vi "RT - Initialize Valves.vi"(8 "error in":errorcluster) -> (0 "error out":errorcluster)   [LabVIEW 2018]
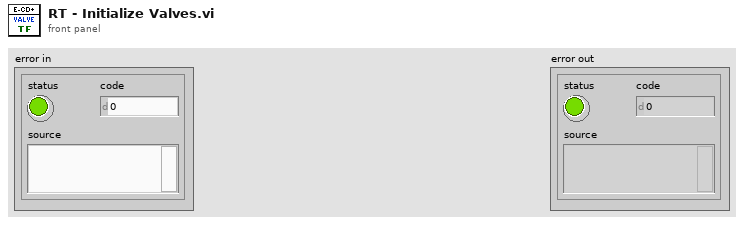
[diagram p1: front panel]
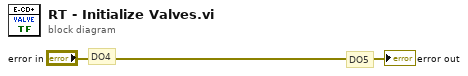
[diagram p0: block diagram]
diagram:
  # "DO5"
  # "DO4"
  "error out" <- "error in"
